vi "Move Group Along An Arc.vi"(4 "error in (no error)":errorcluster, 5 "Arc  Parameters":T1 {"arc sweep angle (0 degrees)" format="%.6g"; "Second coordonate of arc center (0 units)" format="%.6g"; "first coordonate of arc center (0 units)" format="%.6g"}, 6 "Group Number (1)":i32=1 min=1, 7 "VISA resource name":refnum<visa-resource-name>) -> (0 "error out":errorcluster, 3 "VISA resource name out":refnum<visa-resource-name>)   [LabVIEW 2019, in "Newport ESP301.lvlib"]
doc: "This command initiates motion of a group along an arc. It causes all axes assigned to the group to move with predefined vectorial (tangential) velocity, acceleration and deceleration along an arc. The group target position is determined based on the position of axes at the beginning of move, center of arc and sweep angle.\nIf this command is received while a group move is in progress, the new command gets enqueued into a “via point” buffer. Please refer to Advanced Capabilities section for a detailed description of via point buffer implementation. The enqueued commands get executed on a FIFO basis when the move already in progress has reached its destination. The group does not come to a stop at the end of last move. Instead, there will be a smooth transition to the new move command, just as if it were one compound move (combination of multiple moves).\n<B>Note:</B> Only trapezoid velocity profile is employed linear interpolation motion.\n<B>Note:</B> The transition from last move to new move will be smooth if tangential velocity at the end of last move is the same as that at the beginning of new move."
uses:
  Newport ESP301.lvlib
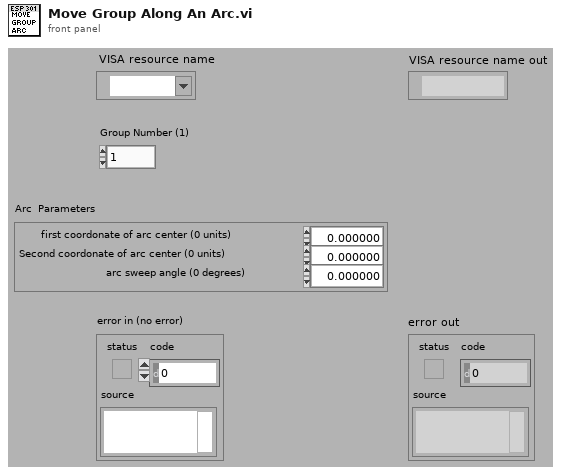
[diagram p1: front panel]
types:
  T1 = cluster{"first coordonate of arc center (0 units)":dbl, "Second coordonate of arc center (0 units)":dbl, "arc sweep angle (0 degrees)":dbl}
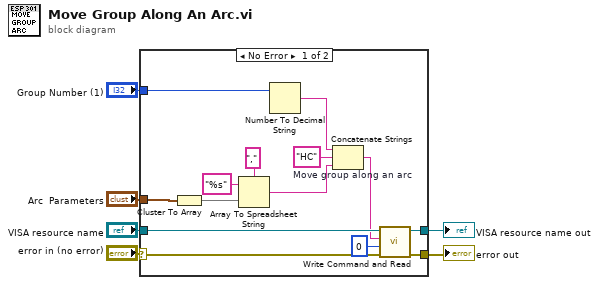
[diagram p0: block diagram]
diagram:
  n1 = case shown="No Error" "error in (no error)" {
    selector: "error in (no error)" -> [w17 w22]
    tunnel: [w19 w22] -> w6
    tunnel: "VISA resource name" -> [w20 w21]
    tunnel: [w18 w21] -> w5
    tunnel: "Group Number (1)" -> [w13 _]
    tunnel: "Arc  Parameters" -> [w9 _]
    frame No Error {
      w16 = "HC"  # Move group along an arc
      n2 = Cluster To Array(cluster=w9) -> (array=w10:dbl[])
      n3 = Array To Spreadsheet String(delimiter (Tab)="," ("séparateur (Tabulation)"), array=w10, 3:"%s" ("chaîne de format")) -> (spreadsheet string=w11:string)
      n4 = Number To Decimal String(number=w13) -> (decimal integer string=w15:string)  [unwired: 1 in]
      n5 = Concatenate Strings(w15, w16, w11) -> (w14:string)
      n6 = call "Write Command and Read.vi"("error in (no error)"=w17, "Bytes to read (100)"=u32 0, "Command"=w14, "VISA resource name"=w20) -> ("error out"=w19:errorcluster, "VISA resource name out"=w18:refnum<visa-resource-name>)  [unwired: 3 in, 1 out]
    }
    frame Error {
    }
  }
  "error out" <- w6
  "VISA resource name out" <- w5
